vi "ConvertBlockDiagram.vi"(5 "Source Directory":path, 6 "error in":errorcluster, 9 "VI Interpreter":refnum<class "VI Interpreter.lvclass">) -> (0 "error out":errorcluster, 3 "VI Interpreter out":refnum<class "VI Interpreter.lvclass">)   [LabVIEW 2014, in "PythonBDConverter.lvclass"]
uses:
  PythonBDConverter.lvclass
  Parsing/Python Functions.lvlib
  VI Interpreter/Classes/VI Interpreter/VI Interpreter.lvclass
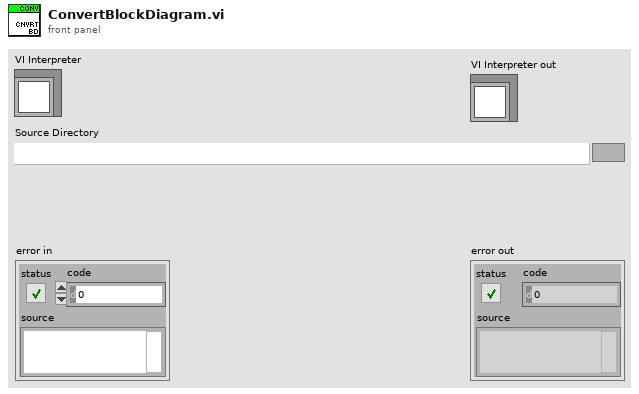
[diagram p1: front panel]
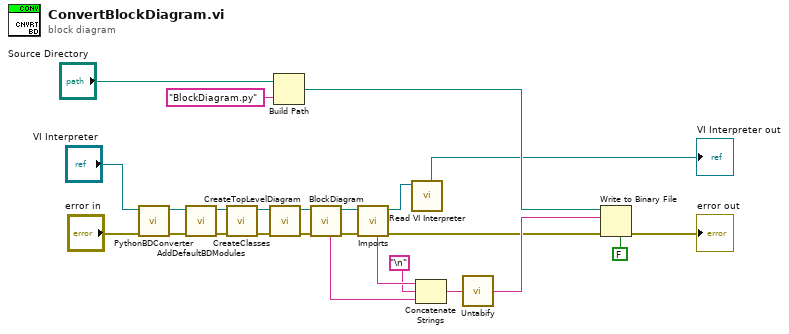
[diagram p0: block diagram]
diagram:
  n1 = call "PythonBDConverter.vi"("error in"="error in", "VI Interpreter in"="VI Interpreter") -> ("error out"=w18:errorcluster, "PythonConverter out"=w19:refnum<class "PythonBDConverter.lvclass">)  [unwired: 6 in]
  n2 = call "AddDefaultBDModules.vi"("error in"=w18, "PythonConverter in"=w19) -> ("error out"=w16:errorcluster, "PythonConverter out"=w17:refnum<class "PythonBDConverter.lvclass">)  [unwired: 6 in]
  n3 = call "CreateClasses.vi"("error in"=w16, "PythonConverter in"=w17) -> ("error out"=w14:errorcluster, "PythonConverter out"=w15:refnum<class "PythonBDConverter.lvclass">)  [unwired: 8 in]
  n4 = call "CreateTopLevelDiagram.vi"("error in"=w14, "PythonConverter in"=w15) -> ("error out"=w25:errorcluster, "PythonConverter out"=w13:refnum<class "PythonBDConverter.lvclass">)  [unwired: 8 in]
  n5 = Build Path(base path="Source Directory", name or relative path="BlockDiagram.py" ("string")) -> (appended path=w21:path)
  n6 = call "BlockDiagram.vi"("error in"=w25, "PythonConverter in"=w13) -> ("error out"=w11:errorcluster, "PythonConverter out"=w12:refnum<class "PythonBDConverter.lvclass">, "BlockDiagram"=w23:string)  [unwired: 5 in]
  n7 = call "Imports.vi"("error in"=w11, "PythonConverter in"=w12) -> ("error out"=w4:errorcluster, "PythonConverter out"=w3:refnum<class "PythonBDConverter.lvclass">, "imports"=w24:string)  [unwired: 5 in]
  n8 = call "Read VI Interpreter.vi"("PythonConverter_BD in"=w3) -> ("VI Interpreter"=→"VI Interpreter out":refnum<class "VI Interpreter.lvclass">)  [unwired: 7 in, 1 out]
  n9 = Concatenate Strings(w24, "\n", w23) -> (w20:string)
  n10 = call "Untabify.vi"("string in"=w20) -> ("string out"=w7:string)  [unwired: 1 in]
  n11 = Write to Binary File(file (use dialog)=w21, data=w7, error in=w4, 5:FALSE ("prepend array or string size? (T)")) -> (error out=→"error out":errorcluster)  [unwired: 2 in, 2 out]
